vi "is_index_in_list.vi"(8 "t2":i32, 9 "t1":i32, 10 "t0":i32, 11 "check index":i32) -> (3 "result":bool)   [LabVIEW 2020]
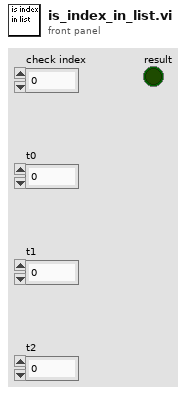
[diagram p1: front panel]
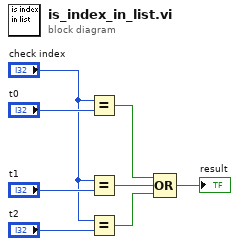
[diagram p0: block diagram]
diagram:
  n1 = Equal?(x="check index", y="t0") -> (x = y?=w4:bool)
  n2 = Equal?(x="check index", y="t1") -> (x = y?=w3:bool)
  n3 = Equal?(x="check index", y="t2") -> (x = y?=w2:bool)
  n4 = Compound Arithmetic op=OR(w4, w3, w2) -> (→"result":bool)
